vi "Write I16.vi"(8 "Error In":errorcluster, 10 "Value":i16, 11 "Writer In":refnum<class "Writer.lvclass">) -> (0 "Error Out":errorcluster, 3 "Writer Out":refnum<class "Writer.lvclass">)   [LabVIEW 2017, in "LabPack.lvlib" / "Writer.lvclass"]
doc: "Writes and encodes a signed 16-bit integer to the MessagePack binary data format."
uses:
  Writer.lvclass
  Writer.lvclass/Writer.ctl
  Status/Read Is Error.vi
  Status/Read Status.vi
  Status/Read Status Message.vi
  <vilib>/Utility/error.llb/Error Cluster From Error Code.vi
  Utility/Status Code.vi
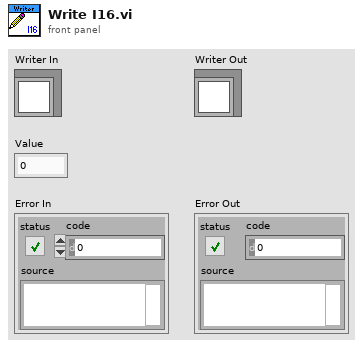
[diagram p1: front panel]
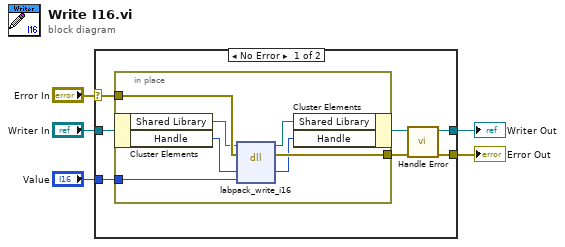
[diagram p0: block diagram]
diagram:
  n1 = case shown="No Error" "Error In" {
    selector: "Error In" -> [w12 w20]
    tunnel: "Writer In" -> [w11 w21]
    tunnel: [w8 w21] -> w3
    tunnel: [w6 w20] -> w2
    tunnel: "Value" -> [w9 _]
    frame No Error {
      n2 = in-place {
        in-place-border: w12 -> [w19]
        in-place-border: [w18] -> w7
        in-place-border: w9 -> [w13]
        n3 = in-place-cluster #1(w11) -> ("Shared Library"=w15:path, "Handle"=w17:u64)
        n4 = dll-call lib="D:/Users/cfield/Code/MessagePack/LabPack/LabVIEW/trunk/src/LabPack/Private/labpack-x64.dll" fn="labpack_write_i16"(path in=w15, error in=w19, "writer"=w17, "value"=w13) -> (path out=w14:path, error out=w18:errorcluster, "writer"=w16:u64)  [unwired: 3 in]
        n5 = in-place-cluster #1("Shared Library"=w14, "Handle"=w16) -> (w10:refnum<class "Writer.lvclass">)
      }
      n6 = call "Handle Error.vi"("Error In"=w7, "Writer In"=w10) -> ("Error Out"=w6:errorcluster, "Writer Out"=w8:refnum<class "Writer.lvclass">)  [unwired: 8 in]
    }
    frame Error {
    }
  }
  "Writer Out" <- w3
  "Error Out" <- w2
